vi "Select Mirror Unit.vi"(8 "error in (no error)":errorcluster {"code" format="%.0x"}, 9 "Mirror Unit Position (1)":i32=1, 10 "Device Number (1)":i32=1, 11 "VISA Resource Name":refnum<visa-resource-name>) -> (0 "error out":errorcluster {"code" format="%.0x"}, 3 "VISA Resource Name Out":refnum<visa-resource-name>)   [LabVIEW 2020, in "Olympus IX BX Series.lvlib"]
doc: "Engages the specified (fluorescence) mirror unit in the light axis.\n\nNotes:\n(1) This VI is valid only for Olympus IX2 model."
uses:
  Olympus IX BX Series.lvlib
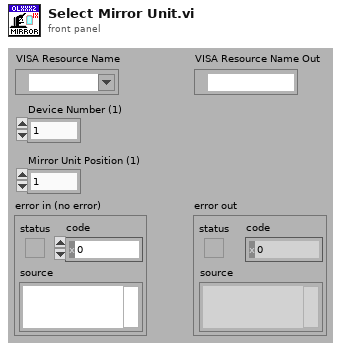
[diagram p1: front panel]
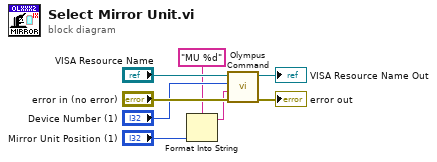
[diagram p0: block diagram]
diagram:
  n1 = Format Into String(format string="MU %d", "Mirror Unit Position (1)") -> (resulting string=w5:string)  [unwired: 2 in, 1 out]
  n2 = call "Olympus Command.vi"("error in (no error)"="error in (no error)", "Command string"=w5, "Device Number (1)"="Device Number (1)", "VISA Resource Name"="VISA Resource Name") -> ("error out"=→"error out":errorcluster, "VISA Resource Name Out"=→"VISA Resource Name Out":refnum<visa-resource-name>)  [unwired: 5 in, 1 out]
